vi "Write to Hardware.vi"(8 "error in":errorcluster, 9 "trigger values":dbl[](array[numeric]), 10 "values":dbl[](array[numeric]), 11 "triggers execution unit":refnum<class "Triggers Execution Unit.lvclass">) -> (0 "error out":errorcluster, 1 "trigger values out":dbl[](array[numeric]), 2 "values out":dbl[](array[numeric]), 3 "triggers execution unit out":refnum<class "Triggers Execution Unit.lvclass">)   [LabVIEW 2020, in "AIM MIL-STD-1553 Engine.lvlib" / "Implementation.lvlib" / "Triggers Execution Unit.lvclass"]
uses:
  Triggers Execution Unit.lvclass
  C:/dev/git/niveristand-aim-milStd1553-custom-device/Source/Custom Device Support/Engine/Implementation/Execution Unit/Execution Unit.lvclass
  Execution Unit/Execution Unit.lvclass/Execution Unit.ctl
  Triggers Execution Unit.lvclass/Triggers Execution Unit.ctl
  Hardware API/AIM MIL-STD-1553 Hardware API.lvlib
  Execution Unit/Execution Unit.lvclass
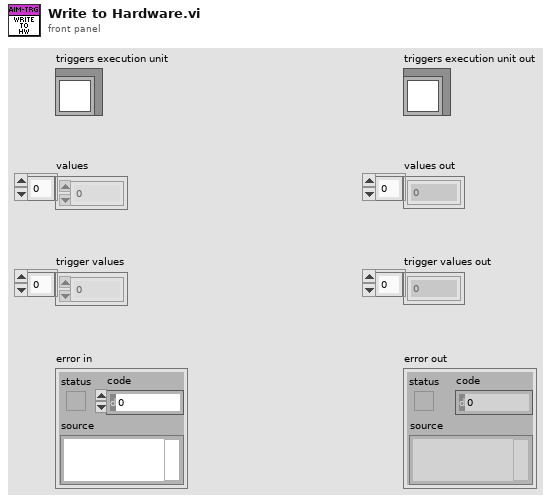
[diagram p1: front panel]
types:
  T1 = typedef "AIM MIL-STD-1553 Hardware API.lvlib/Module Reference.ctl" = u32
  T2 = typedef "Address.ctl" = u16
  T3 = typedef "AIM MIL-STD-1553 Engine.lvlib/Implementation.lvlib/Triggers Execution Unit.lvclass/Triggerable Frame.ctl" = cluster{"Acyclic Transfer IDs":u16[], "Acyclic Messages":T4[]}
  T4 = typedef "AIM MIL-STD-1553 Engine.lvlib/Custom Device.lvlib/Compiled Message.ctl" = cluster{"Message Section Handle":T5, "First Parameter Index":i32, "Parameter Channel Handles":T5[], "Direction":T6, "Parameters":T7[], "Receiving RT Address":u8, "Receiving RT Sub-address":u8, "Transmitting RT Address":u8, "Transmitting RT Sub-address":u8, "Word Count":u8, "Buffer Type":enum16{"unknown", "BC Message Buffer", "RT Message Buffer"}, "Buffer ID":u16, "Terminal Type":enum16{"Bus Controller", "Remote Terminal"}, "Timestamp Enabled":bool, "Timestamp Channel Handle":T5}
  T5 = typedef "Custom Device API.lvlib/Custom Device Item Ref.ctl" = u64
  T6 = typedef "Direction.ctl" = enum16{"Rx", "Tx"}
  T7 = typedef "Parameter Definition.ctl" = cluster{"start index":i32, "size (bits)":i32, "encoding":enum16{"BNR", "BCD", "Discrete"}, "signed":bool, "multiplier":dbl, "offset":dbl}
  T8 = typedef "Running Status.ctl" = enum16{"Running", "Stopped"}
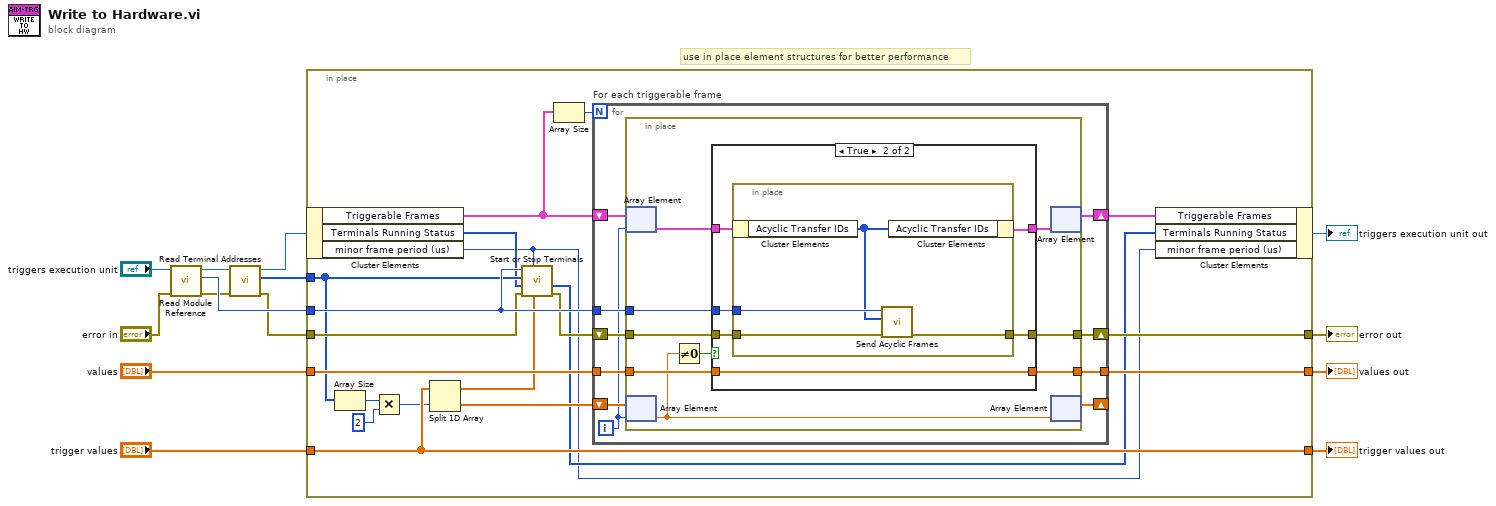
[diagram p0: block diagram]
diagram:
  # "use in place element structures for better performance"
  n1 = call "Read Module Reference.vi"("error in"="error in", "execution unit"="triggers execution unit") -> ("error out"=w1:errorcluster, "module reference"=w8:T1, "execution unit out"=w5:refnum<class "Triggers Execution Unit.lvclass">)  [unwired: 7 in]
  n2 = call-dynamic "Read Terminal Addresses.vi"("error in (no error)"=w1, "Execution Unit in"=w5) -> ("error out"=w3:errorcluster, "terminal addresses"=w2:T2[], "Execution Unit out"=w4:refnum<class "Triggers Execution Unit.lvclass">)  [unwired: 7 in]
  n3 = in-place {
    in-place-border: w3 -> [w21]
    in-place-border: "values" -> [w33]
    in-place-border: "trigger values" -> [w27]
    in-place-border: [w27] -> w12
    in-place-border: [w32] -> w11
    in-place-border: [w31] -> w10
    in-place-border: w8 -> [w22]
    in-place-border: w2 -> [w18]
    n4 = in-place-cluster #1(w4) -> ("Triggerable Frames"=w29:T3[], "Terminals Running Status"=w17:T8[], "minor frame period (us)"=w16:i32)
    n5 = Array Size(array=w18) -> (size(s)=w25:i32)
    n6 = Multiply(x=w25, y=2) -> (x*y=w23:i32)
    n7 = Split 1D Array(array=w27, index=w23) -> (first subarray=w15:dbl[], second subarray=w26:dbl[])
    n8 = call "Start or Stop Terminals.vi"("trigger values"=w15, "minor frame period (us)"=w16, "error in"=w21, "running status"=w17, "terminal addresses"=w18, "Module Handle"=w22) -> ("error out"=w20:errorcluster, "running status out"=w19:T8[])  [unwired: 4 in]
    n9 = Array Size(array=w29) -> (size(s)=w30:i32)
    n10 = for "For each triggerable frame" {
      N: w30 -> [_]
      tunnel: w22 -> [w43]
      tunnel: w33 -> [w41]
      tunnel: [w40] -> w31
      shift-right: [w39] -> w32
      shift-left: w20 -> [w42]
      shift-right: [w35] -> w28
      shift-left: w29 -> [w38]
      shift-right: [w36] -> _
      shift-left: w26 -> [w37]
      i -> [w34]
      n11 = in-place {
        in-place-border: w43 -> [w52]
        in-place-border: w42 -> [w51]
        in-place-border: w41 -> [w50]
        in-place-border: [w49] -> w40
        in-place-border: [w48] -> w39
        n12 = in-place-array #2(w38, w34) -> (w46:T3)
        n13 = in-place-array #3(w37, w34) -> (w44:dbl)
        n14 = Not Equal To 0?(x=w44) -> (x != 0?=w47:bool)
        n15 = case shown="True" w47 {
          tunnel: w52 -> [_ w58]
          tunnel: w46 -> [w53 w57]
          tunnel: w51 -> [w55 w59]
          tunnel: w50 -> [w54 w61]
          tunnel: [w54 w61] -> w49
          tunnel: [w55 w60] -> w48
          tunnel: [w53 w56] -> w45
          frame False {
          }
          frame True {
            n16 = in-place {
              in-place-border: [w65] -> w60
              in-place-border: w59 -> [w64]
              in-place-border: w58 -> [w63]
              n17 = in-place-cluster #4(w57) -> ("Acyclic Transfer IDs"=w62:u16[])
              n18 = call "Send Acyclic Frames.vi"("error in"=w64, "transfer ids"=w62, "module handle"=w63) -> ("error out"=w65:errorcluster)  [unwired: 7 in, 1 out]
              n19 = in-place-cluster #4("Acyclic Transfer IDs"=w62) -> (w56:T3)
            }
          }
        }
        n20 = in-place-array #2(w45) -> (w35:T3[])  [unwired: 1 out]
        n21 = in-place-array #3(w44) -> (w36:dbl[])  [unwired: 1 out]
      }
    }
    n22 = in-place-cluster #1("Triggerable Frames"=w28, "Terminals Running Status"=w19, "minor frame period (us)"=w16) -> (→"triggers execution unit out":refnum<class "Triggers Execution Unit.lvclass">)
  }
  "error out" <- w11
  "values out" <- w10
  "trigger values out" <- w12
